vi "Panel.vi"(11 "Panel in":refnum<class "Panel.lvclass">) -> ()   [LabVIEW 2020, in "OOPanel.lvlib" / "Panel.lvclass"]
uses:
  <vilib>/IlluminatedG/IG OOPanel/OOPanel/Panel/Panel.lvclass
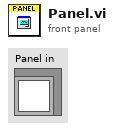
[diagram p1: front panel]
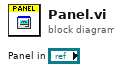
[diagram p0: block diagram]
diagram:
